vi "SingleConnection.vi"() -> ()   [LabVIEW 2016]
doc: "This VI acts as a server for an incoming websockets connection. Receives/sends string data to the connected client.\nWebSockets 1.6.0.22\nSam Sharp - MediaMongrels Ltd\nCopyright (c) 2016, MediaMongrels Ltd"
uses:
  StatusCode.ctl
  <vilib>/Platform/browser.llb/Open URL in Default Browser (path).vi
  WebSockets.lvlib
panel:
  in  "Client Type to Open":enum16{"Web Client", "LabVIEW Client"}(ring)
  out "Status Code":T1=1000 items=["Normal Closure"=1000, "Going Away"=1001, "Protocol Error"=1002, "Wrong Data Type"=1003, "Reserved 1004"=1004, "Reserved 1005"=1005, "Reserved 1006"=1006, "Non Consistent Data Type"=1007, "Policy Violation"=1008, "Message Too Big"=1009, "Extensions Negotiation Error"=1010, "Unexpected Condition"=1011, "Reserved 1015"=1015]
  out "Close Reason":string
  in  "Resource Names":string[](array[string])=["/resource/name"]
  out "Host":string
  out "Resource Name":string
  out "Request URI":string
  out "HTTP Headers":variant
  in  "Stop":bool
  out "Received Data":string
  in  "Send":bool
  in  "Data":string
  # "WebSockets Example Server"
  # "This VI is a simple example of sending/receiving data using WebSockets.\nIt waits for a single incoming WebSockets connection on Port 6123 and\nthen displays incoming string data. Strings can also be sent back to the client.\n\nInstructions for use:\n1) Run this VI\n2) Open the index.html file located in the examples folder\n3) The index.html will display the status of the connection and once established, data can be sent/received from either this VI or the index.html file."
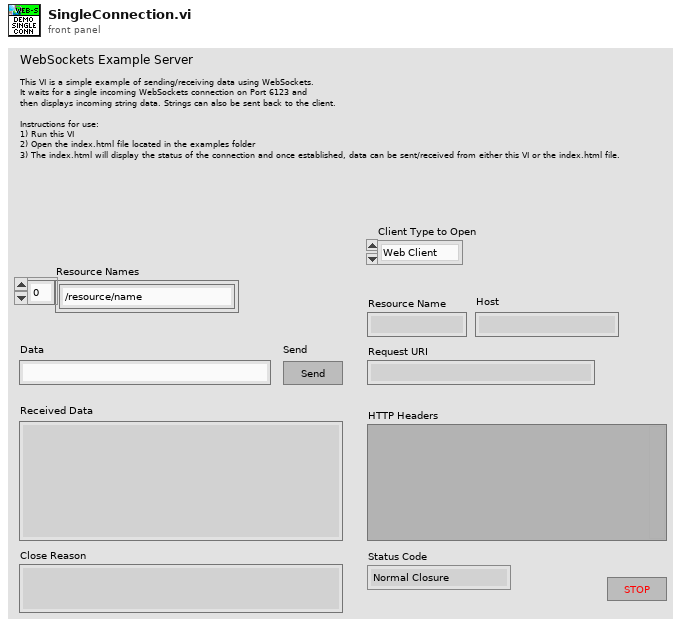
[diagram p1: front panel]
types:
  T1 = typedef "WebSockets.lvlib/StatusCode.ctl" = u16
  T2 = typedef "WebSockets.lvlib/Opcode.ctl" = enum8{"Continuation Frame", "Text Frame", "Binary Frame", "Reserved 3", "Reserved 4", "Reserved 5", "Reserved 6", "Reserved 7", "Connection Close", "Ping", "Pong", "Reserved B", "Reserved C", "Reserved D", "Reserved F"}
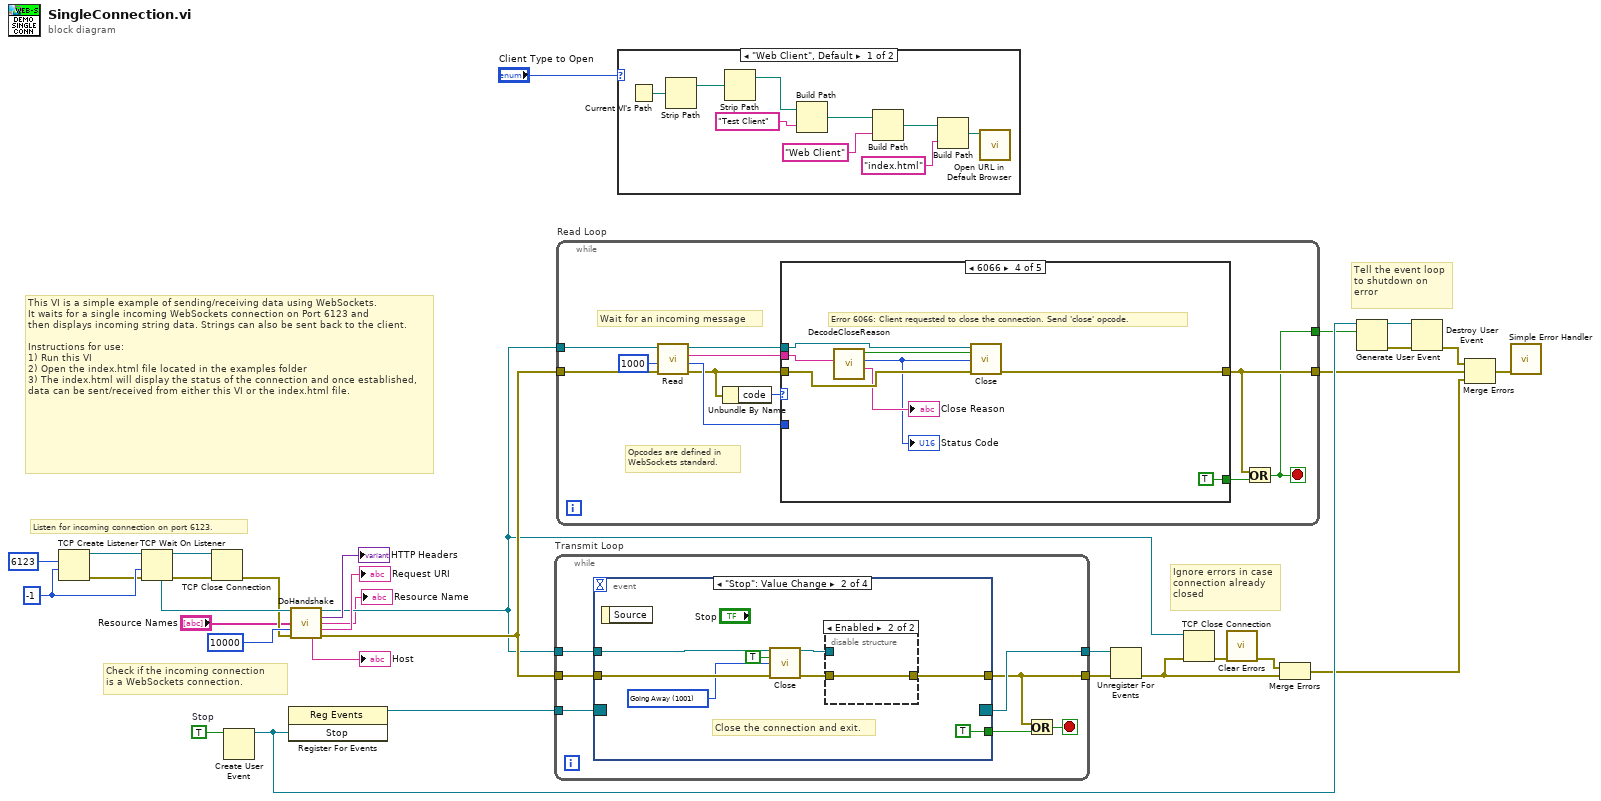
[diagram p0: block diagram]
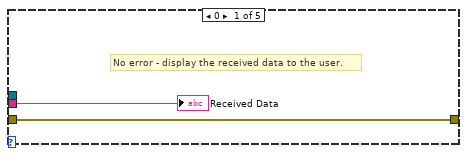
[diagram p3: hidden frame]
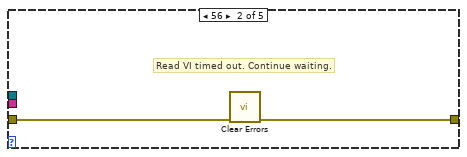
[diagram p4: hidden frame]
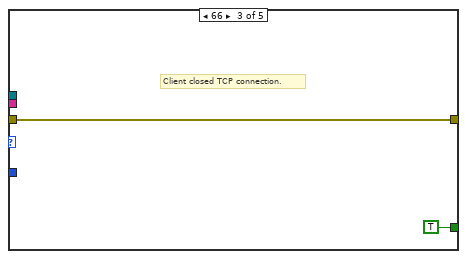
[diagram p5: hidden frame]
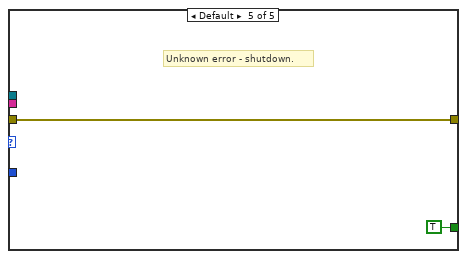
[diagram p6: hidden frame]
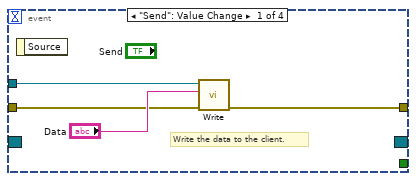
[diagram p7: hidden frame]
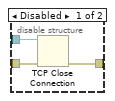
[diagram p8: hidden frame]
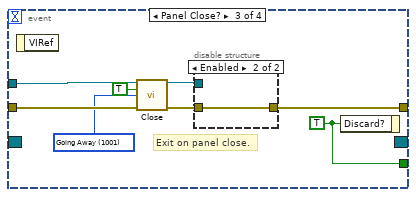
[diagram p9: hidden frame]
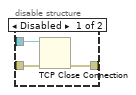
[diagram p10: hidden frame]
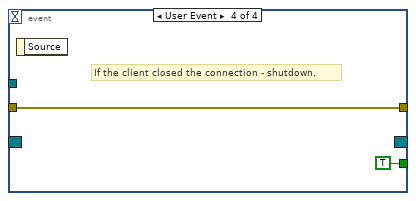
[diagram p11: hidden frame]
diagram:
  w24 = TRUE  # Stop
  w31 = -1 ("timeout ms (25000)")
  # "Ignore errors in case\nconnection already\nclosed"
  # "Tell the event loop to shutdown on error"
  # "This VI is a simple example of sending/receiving data using WebSockets.\nIt waits for a single incoming WebSockets connection on Port 6123 and\nthen displays incoming string data. Strings can also be sent back to the client.\n\nInstructions for use:\n1) Run this VI\n2) Open the index.html file located in the examples folder\n3) The index.html will display the status of the connection and once established, data can be sent/received from either this VI or the index.html file."
  # "Check if the incoming connection\nis a WebSockets connection."
  # "Listen for incoming connection on port 6123."
  n1 = TCP Create Listener(9:w31, 10:u16 6123 ("port")) -> (0:w29:errorcluster, 3:w30:refnum<k5>)  [unwired: 3 in, 1 out]
  n2 = TCP Wait On Listener(8:w29, 9:w31, 11:w30) -> (0:w26:errorcluster, 3:w27:refnum<k5>, 4:w28:refnum<k5>)  [unwired: 1 in, 2 out]
  n3 = TCP Close Connection(connection ID=w27, error in (no error)=w26) -> (error out=w4:errorcluster)  [unwired: 1 in, 1 out]
  n4 = Create User Event(user event datatype=w24) -> (user event=w22:refnum<user-event>)  [unwired: 1 in, 1 out]
  n5 = register-events(w22) -> (reference out=w25:refnum<event-registration>)  [unwired: 2 in, 1 out]
  n6 = call "DoHandshake.vi"("WebSocket Connection in"=w28, "Resource Names"="Resource Names", "timeout ms (5000)"=10000 ("timeout ms (25000)"), "error in (no error)"=w4) -> ("WebSocket Connection out"=w10:refnum<k5>, "Headers Out"=→"HTTP Headers":variant, "Resource Name"=→"Resource Name":string, "Request URI"=→"Request URI":string, "Host"=→"Host":string, "error out"=w12:errorcluster)  [unwired: 6 in]
  n7 = while "Transmit Loop" {
    tunnel: w10 -> [w39]
    tunnel: w25 -> [w38]
    tunnel: [w37] -> w23
    tunnel: [w33] -> w13
    tunnel: w12 -> [w36]
    stop <- w34 stop-if-true
    n8 = event shown="[1] \"Stop\": Value Change" {
      selector: w38 -> [_ _ _ _]
      dyn-events: [_ _ _ _] -> w37
      timeout: _ -> [_ _ _ _]
      tunnel: w39 -> [w43 w50 w63 _]
      tunnel: [_ TRUE w61 TRUE] -> w35
      tunnel: [w40 w48 w59 w68] -> w33
      tunnel: w36 -> [w41 w46 w58 w68]
      event "Send": Value Change {
        # "Write the data to the client."
        n9 = event-data() -> ()  [unwired: 1 in, 1 out]
        n10 = call "Write.vi"("error in (no error)"=w41, "Data"="Data", "WebSocket Connection in"=w43) -> ("error out"=w40:errorcluster)  [unwired: 7 in, 1 out]
      }
      event "Stop": Value Change {
        w45 = T1 1001 items=["Normal Closure"=1000, "Going Away"=1001, "Protocol Error"=1002, "Wrong Data Type"=1003, "Reserved 1004"=1004, "Reserved 1005"=1005, "Reserved 1006"=1006, "Non Consistent Data Type"=1007, "Policy Violation"=1008, "Message Too Big"=1009, "Extensions Negotiation Error"=1010, "Unexpected Condition"=1011, "Reserved 1015"=1015] ("Status Code")
        # "Close the connection and exit."
        n11 = event-data() -> ()  [unwired: 1 in, 1 out]
        n12 = call "Close.vi"("WebSocket Connection in"=w50, "Send Reason (F)"=TRUE, "Status Code"=w45, "error in (no error)"=w46) -> ("WebSocket Connection in"=w49:refnum<k5>, "error out"=w47:errorcluster)  [unwired: 10 in]
        n13 = disable-structure shown="Enabled" {
          disable-tunnel: w49 -> [w54 _]
          disable-tunnel: [w53 w55] -> w48
          disable-tunnel: w47 -> [w52 w55]
          frame Disabled {
            n14 = TCP Close Connection(connection ID=w54, error in (no error)=w52) -> (error out=w53:errorcluster)  [unwired: 1 in, 1 out]
          }
          frame Enabled {
          }
        }
      }
      event Panel Close? {
        w57 = T1 1001 items=["Normal Closure"=1000, "Going Away"=1001, "Protocol Error"=1002, "Wrong Data Type"=1003, "Reserved 1004"=1004, "Reserved 1005"=1005, "Reserved 1006"=1006, "Non Consistent Data Type"=1007, "Policy Violation"=1008, "Message Too Big"=1009, "Extensions Negotiation Error"=1010, "Unexpected Condition"=1011, "Reserved 1015"=1015] ("Status Code")
        w61 = TRUE ("Discard?")
        # "Exit on panel close."
        n15 = event-data() -> ()  [unwired: 1 in, 1 out]
        n16 = call "Close.vi"("WebSocket Connection in"=w63, "Send Reason (F)"=TRUE, "Status Code"=w57, "error in (no error)"=w58) -> ("WebSocket Connection in"=w62:refnum<k5>, "error out"=w60:errorcluster)  [unwired: 10 in]
        n17 = disable-structure shown="Enabled" {
          disable-tunnel: w62 -> [w66 _]
          disable-tunnel: w60 -> [w65 w67]
          disable-tunnel: [w64 w67] -> w59
          frame Disabled {
            n18 = TCP Close Connection(connection ID=w66, error in (no error)=w65) -> (error out=w64:errorcluster)  [unwired: 1 in, 1 out]
          }
          frame Enabled {
          }
        }
        n19 = event-data("Discard?"=w61) -> ()  [unwired: 1 in, 1 out]
      }
      event User Event {
        # "If the client closed the connection - shutdown."
        n20 = event-data() -> ()  [unwired: 1 in, 1 out]
      }
    }
    n21 = Or(x=w33, y=w35) -> (x .or. y?=w34:bool)
  }
  n22 = while "Read Loop" {
    tunnel: w10 -> [w80]
    tunnel: [w70] -> w21
    tunnel: [w72] -> w11
    tunnel: w12 -> [w73]
    stop <- w70 stop-if-true
    # "Wait for an incoming message"
    # "Opcodes are defined in\nWebSockets standard."
    n23 = call "Read.vi"("error in (no error)"=w73, "timeout ms (5000)"=1000 ("timeout ms (25000)"), "WebSocket Connection in"=w80) -> ("error out"=w74:errorcluster, "Opcode out"=w75:T2, "Data"=w77:string, "WebSocket Connection out"=w76:refnum<k5>)  [unwired: 5 in]
    n24 = Unbundle By Name(w74) -> ("code"=w78:i32)
    n25 = case shown="6066" w78 {
      tunnel: w77 -> [w82 _ _ w90 _]
      tunnel: [_ _ TRUE TRUE TRUE] -> w71
      tunnel: w76 -> [_ _ _ w94 _]
      tunnel: w75 -> [_ _ _ _ _]
      tunnel: w74 -> [w81 w84 w85 w92 w95]
      tunnel: [w81 w83 w85 w91 w95] -> w72
      frame 0 {
        # "No error - display the received data to the user."
        "Received Data" <- w82
      }
      frame 56 {
        # "Read VI timed out. Continue waiting."
        n26 = call <vilib>:"Clear Errors.vi"("error in (no error)"=w84) -> ("error out"=w83:errorcluster)  [unwired: 5 in, 1 out]
      }
      frame 66 {
        # "Client closed TCP connection."
      }
      frame 6066 {
        # "Error 6066: Client requested to close the connection. Send 'close' opcode."
        n27 = call "DecodeCloseReason.vi"("Data"=w90) -> ("Reason"=→"Close Reason":string, "Status Code"=w88:T1, "Close Reason Given"=w87:bool)  [unwired: 8 in]
        "Status Code" <- w88
        n28 = call "Close.vi"("WebSocket Connection in"=w94, "Send Reason (F)"=w87, "Status Code"=w88, "error in (no error)"=w92) -> ("error out"=w91:errorcluster)  [unwired: 10 in, 1 out]
      }
      frame Default {
        # "Unknown error - shutdown."
      }
    }
    n29 = Or(x=w72, y=w71) -> (x .or. y?=w70:bool)
  }
  n30 = case shown="\"Web Client\", Default" "Client Type to Open" {
    frame "Web Client", Default {
      n31 = Current VI's Path() -> (path=w105:path)
      n32 = Strip Path(path=w105) -> (stripped path=w104:path)  [unwired: 1 out]
      n33 = Strip Path(path=w104) -> (stripped path=w103:path)  [unwired: 1 out]
      n34 = Build Path(base path=w103, name or relative path="Test Client") -> (appended path=w100:path)
      n35 = Build Path(base path=w100, name or relative path="Web Client") -> (appended path=w99:path)
      n36 = Build Path(base path=w99, name or relative path="index.html") -> (appended path=w101:path)
      n37 = call-poly <vilib>:"Open URL in Default Browser.vi"("path"=w101) -> ()  [unwired: 5 in, 2 out]
    }
    frame "LabVIEW Client" {
    }
  }
  n38 = Unregister For Events(event registration refnum=w23, error in=w13) -> (error out=w8:errorcluster)
  n39 = TCP Close Connection(connection ID=w10, error in (no error)=w8) -> (error out=w9:errorcluster)  [unwired: 1 in, 1 out]
  n40 = call <vilib>:"Clear Errors.vi"("error in (no error)"=w9) -> ("error out"=w6:errorcluster)  [unwired: 5 in, 1 out]
  n41 = Merge Errors(w6, w8) -> (w7:errorcluster)
  n42 = Generate User Event(user event=w22, event data cluster=w21) -> (user event out=w20:refnum<user-event>, error out=w19:errorcluster)  [unwired: 2 in]
  n43 = Destroy User Event(user event=w20, error in=w19) -> (error out=w18:errorcluster)
  n44 = Merge Errors(w18, w11, w7) -> (w14:errorcluster)
  n45 = call <vilib>:"Simple Error Handler.vi"("error in (no error)"=w14) -> ()  [unwired: 4 in, 5 out]
